vi "Destination Room Position.vi"(11 "Amphipod Type":string) -> (3 "Destination Room Position":i32)   [LabVIEW 2019, in "23.lvlib" / "State.lvclass"]
uses:
  State.lvclass
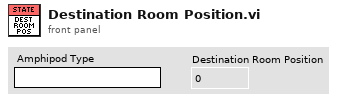
[diagram p1: front panel]
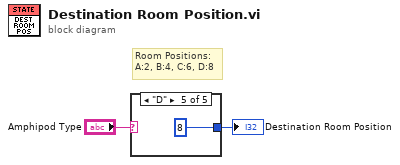
[diagram p0: block diagram]
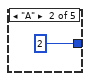
[diagram p3: hidden frame]
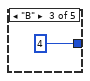
[diagram p4: hidden frame]
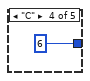
[diagram p5: hidden frame]
diagram:
  # "Room Positions:\nA:2, B:4, C:6, D:8"
  n1 = case shown="\"D\"" "Amphipod Type" {
    tunnel: [_ 2 4 6 8] -> w2
    frame Default {
    }
    frame "A" {
    }
    frame "B" {
    }
    frame "C" {
    }
    frame "D" {
    }
  }
  "Destination Room Position" <- w2
